vi "TypesetInsideMathmode.vi"(8 "Needs $$?":bool=TRUE, 11 "DirtyString":string) -> (0 "ChosenStringtype":string, 2 "Mathmode String":string, 3 "De-dollared String":string)   [LabVIEW 2018]
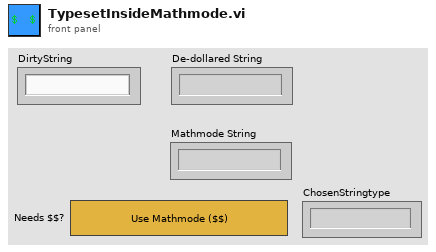
[diagram p1: front panel]
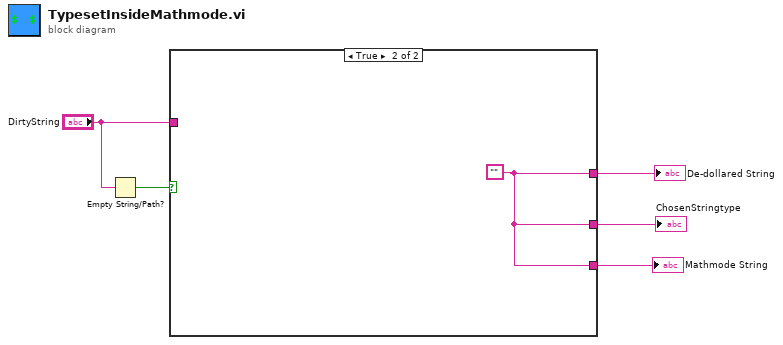
[diagram p0: block diagram]
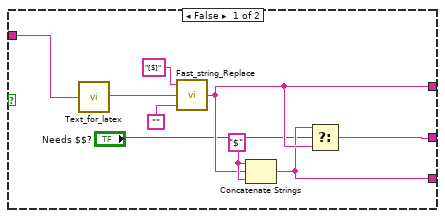
[diagram p2: hidden frame]
diagram:
  n1 = Empty String/Path?(string/path="DirtyString") -> (empty?=w1:bool)
  n2 = case shown="True" w1 {
    tunnel: [w10 w15] -> w5
    tunnel: [w9 w15] -> w4
    tunnel: [w7 w15] -> w3
    tunnel: "DirtyString" -> [w6 _]
    frame False {
      w11 = "$" ("string")
      n3 = call "Text_for_latex.vi"("Input String"=w6) -> ("Output String"=w12:string)
      n4 = call "Fast_string_Replace.vi"("Replace match with:"="", "Input String"=w12, "regular expression"="[$]") -> ("Output String"=w10:string)  [unwired: 2 out]
      n5 = Concatenate Strings(w11, w10, w11) -> (w9:string)
      n6 = Select(t=w9, s="Needs $$?", f=w10) -> (s? t:f=w7:string)
    }
    frame True {
      w15 = ""
    }
  }
  "De-dollared String" <- w5
  "Mathmode String" <- w4
  "ChosenStringtype" <- w3
